vi "Load PIC and XML.vi"(0 "selected path":path) -> ()   [LabVIEW 2010]
uses:
  <vilib>/Utility/config.llb/Read Key (Path).vi
  <vilib>/Utility/config.llb/NI_LVConfig.lvlib
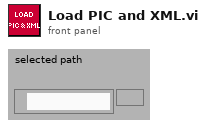
[diagram p1: front panel]
types:
  T1 = typedef "NI_LVConfig.lvlib/Config Data RefNum.ctl" = refnum<k1>
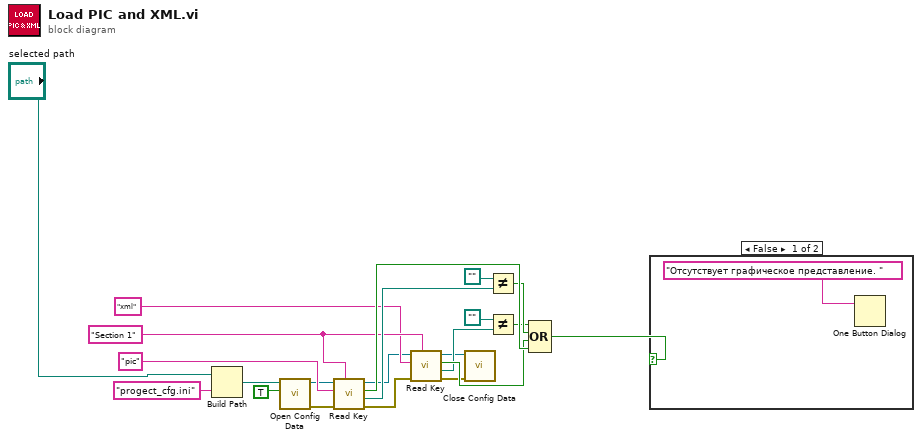
[diagram p0: block diagram]
diagram:
  w12 = "Section 1" ("section")
  n1 = Build Path(base path="selected path", name or relative path="progect_cfg.ini") -> (appended path=w2:path)
  n2 = call <vilib>:"Open Config Data.vi"("create file if necessary (T)"=TRUE, "configuration file path"=w2) -> ("error out"=w4:errorcluster, "refnum"=w5:T1)  [unwired: 7 in, 1 out]
  n3 = call-poly <vilib>:"Read Key.vi"("section"=w12, "error in (no error)"=w4, "key"="pic", "refnum"=w5) -> ("error out"=w8:errorcluster, "value"=w17:path, "found?"=w21:bool, "refnum out"=w7:T1)  [unwired: 4 in]
  n4 = call-poly <vilib>:"Read Key.vi"("section"=w12, "error in (no error)"=w8, "key"="xml", "refnum"=w7) -> ("error out"=w10:errorcluster, "value"=w15:path, "found?"=w20:bool, "refnum out"=w9:T1)  [unwired: 4 in]
  n5 = call <vilib>:"Close Config Data.vi"("error in (no error)"=w10, "refnum"=w9) -> ()  [unwired: 8 in, 2 out]
  n6 = Not Equal?(x=path "", y=w17) -> (x != y?=w19:bool)
  n7 = Not Equal?(x=path "", y=w15) -> (x != y?=w18:bool)
  n8 = Compound Arithmetic op=OR(w18, w19, w20, w21) -> (w22:bool)
  n9 = case shown="False" w22 {
    frame False {
      n10 = One Button Dialog(message="Отсутствует графическое представление. ") -> ()  [unwired: 1 in, 1 out]
    }
    frame True {
      # "Добавить считывание"
    }
  }
